vi "SplitterPowerCheckSingle.vi"(3 "error in (no error)":errorcluster, 5 "Select SG Freq GHz":dbl=2.809 format="%#.5f") -> (0 "error out":errorcluster, 1 "String_PSG_Amp_Split":string, 2 "dBAvg SigGen Power to splitter (dBm)":dbl format="%#.5f", 4 "dBAvg Power Meter Noise Floor (dBm)":dbl format="%#.5f", 6 "dBSSD SigGen Power to splitter (dB)":dbl format="%#.6f")   [LabVIEW 2009]
doc: "Measure SigGen power at splitter including AMP and attenuation switching using N1911A"
panel:
  out "dBPeakToAver (dB)":dbl format="%.5f"
  in  "Select_Interval_between_readings mS":i32=50 min=1 max=1000 step=1
  out "LinAvg SigGen Power to splitter (dBm)":dbl format="%.5f"
  in  "Select NreadingsFromPwrMeterToAverage":i32=10 min=1 max=1000 step=1
  # "Insure that the correct power meter averaging mode is set up prior to this call."
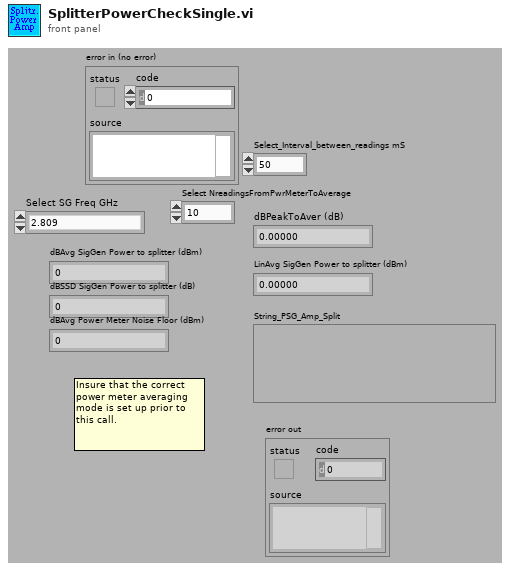
[diagram p1: front panel]
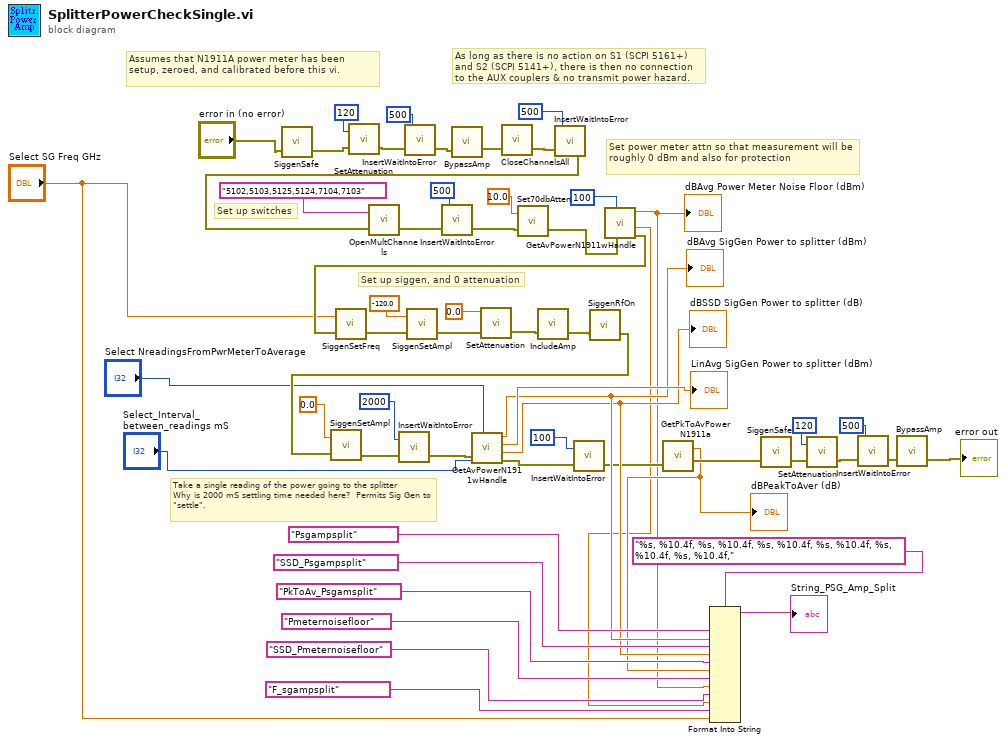
[diagram p0: block diagram]
diagram:
  # "As long as there is no action on S1 (SCPI 5161+) and S2 (SCPI 5141+), there is then no connection to the AUX couplers & no transmit power hazard."
  # "Assumes that N1911A power meter has been setup, zeroed, and calibrated before this vi."
  # "Set power meter attn so that measurement will be roughly 0 dBm and also for protection"
  # "Set up switches"
  # "Take a single reading of the power going to the splitter\nWhy is 2000 mS settling time needed here?  Permits Sig Gen to \"settle\"."
  # "Set up siggen, and 0 attenuation"
  n1 = call "SiggenSafe.vi"("error in (no error)"="error in (no error)") -> ("error out"=w37:errorcluster)  [unwired: 2 in]
  n2 = call "SetAttenuation.vi"("error in (no error)"=w37, "Attenuation (dB)"=120) -> ("error out"=w33:errorcluster)  [unwired: 1 in]
  n3 = call "InsertWaitIntoError.vi"("error in (no error)"=w33, "Wait (msecs)"=500) -> ("error out"=w34:errorcluster)  [unwired: 1 in]
  n4 = call "BypassAmp.vi"("error in (no error)"=w34) -> ("error out"=w36:errorcluster)  [unwired: 2 in]
  n5 = call "CloseChannelsAll.vi"("error in (no error)"=w36) -> ("error out"=w53:errorcluster)  [unwired: 2 in]
  n6 = call "InsertWaitIntoError.vi"("error in (no error)"=w53, "Wait (msecs)"=500) -> ("error out"=w44:errorcluster)  [unwired: 1 in]
  n7 = call "OpenMultChannels.vi"("error in (no error)"=w44, "Channels to be opened"="5102,5103,5125,5124,7104,7103") -> ("error out"=w26:errorcluster)  [unwired: 1 in]
  n8 = call "InsertWaitIntoError.vi"("error in (no error)"=w26, "Wait (msecs)"=500) -> ("error out"=w25:errorcluster)  [unwired: 1 in]
  n9 = call "Set70dbAtten.vi"("error in (no error)"=w25, "Attenuation (dB)"=10.0) -> ("error out"=w9:errorcluster)  [unwired: 1 in]
  n10 = call "GetAvPowerN1911wHandle.vi"("error in (no error)"=w9, "NreadingsFromPwrMeter"=100) -> ("Error out"=w8:errorcluster, "VI dBSSD Power (dB)"=w3:dbl, "VI dBMean Power (dBm)"=w2:dbl)  [unwired: 3 in, 4 out]
  "dBAvg Power Meter Noise Floor (dBm)" <- w2
  n11 = call "SiggenSetFreq.vi"("error in (no error)"=w8, "Freq request (GHz)"="Select SG Freq GHz") -> ("Error status"=w51:errorcluster)  [unwired: 1 out]
  n12 = call "SiggenSetAmpl.vi"("error in (no error)"=w51, "Amplitude request (dBm)"=-120.0) -> ("error out"=w50:errorcluster)  [unwired: 1 out]
  n13 = call "SetAttenuation.vi"("error in (no error)"=w50, "Attenuation (dB)"=0.0) -> ("error out"=w47:errorcluster)  [unwired: 1 in]
  n14 = call "IncludeAmp.vi"("error in (no error)"=w47) -> ("error out"=w46:errorcluster)  [unwired: 2 in]
  n15 = call "SiggenRfOn.vi"("error in (no error)"=w46) -> ("error out"=w45:errorcluster)  [unwired: 2 in]
  n16 = call "SiggenSetAmpl.vi"("error in (no error)"=w45, "Amplitude request (dBm)"=0.0) -> ("error out"=w39:errorcluster)  [unwired: 1 out]
  n17 = call "InsertWaitIntoError.vi"("error in (no error)"=w39, "Wait (msecs)"=2000) -> ("error out"=w40:errorcluster)  [unwired: 1 in]
  n18 = call "GetAvPowerN1911wHandle.vi"("error in (no error)"=w40, "NreadingsFromPwrMeter"="Select NreadingsFromPwrMeterToAverage", "IntervalBetweenReadings (mS)"="Select_Interval_between_readings mS") -> ("Error out"=w11:errorcluster, "VI dBSSD Power (dB)"=w18:dbl, "Computed LinMean Power (dBm)"=→"LinAvg SigGen Power to splitter (dBm)":dbl, "VI dBMean Power (dBm)"=w19:dbl)  [unwired: 2 in, 3 out]
  "dBAvg SigGen Power to splitter (dBm)" <- w19
  "dBSSD SigGen Power to splitter (dB)" <- w18
  n19 = call "InsertWaitIntoError.vi"("error in (no error)"=w11, "Wait (msecs)"=100) -> ("error out"=w10:errorcluster)  [unwired: 1 in]
  n20 = call "GetPkToAvPowerN1911a.vi"("error in (no error)"=w10) -> ("Error out"=w15:errorcluster, "Power returned (dBm)"=w13:dbl)  [unwired: 1 in]
  "dBPeakToAver (dB)" <- w13
  n21 = Format Into String(format string="%s, %10.4f, %s, %10.4f, %s, %10.4f, %s, %10.4f, %s, %10.4f, %s, %10.4f,", "Psgampsplit", w19, "SSD_Psgampsplit", w18, "PkToAv_Psgamsplit", w13, "Pmeternoisefloor", w2, "SSD_Pmeternoisefloor", w3, "F_sgampsplit", "Select SG Freq GHz") -> (resulting string=→"String_PSG_Amp_Split":string)  [unwired: 2 in, 1 out]
  n22 = call "SiggenSafe.vi"("error in (no error)"=w15) -> ("error out"=w29:errorcluster)  [unwired: 2 in]
  n23 = call "SetAttenuation.vi"("error in (no error)"=w29, "Attenuation (dB)"=120) -> ("error out"=w30:errorcluster)  [unwired: 1 in]
  n24 = call "InsertWaitIntoError.vi"("error in (no error)"=w30, "Wait (msecs)"=500) -> ("error out"=w28:errorcluster)  [unwired: 1 in]
  n25 = call "BypassAmp.vi"("error in (no error)"=w28) -> ("error out"=→"error out":errorcluster)  [unwired: 2 in]
